vi "Write OCP Delay.vi"(8 "error in":errorcluster, 10 "Delay":dbl, 11 "3300 in":refnum<class "3300.lvclass">) -> (0 "error out":errorcluster, 3 "3300 out":refnum<class "3300.lvclass">)   [LabVIEW 2019, in "3300.lvlib" / "3300.lvclass"]
uses:
  Library/3300.lvclass
  builds/Instruments/Electronic Load.lvlibp/Library/Electronic Load.lvclass
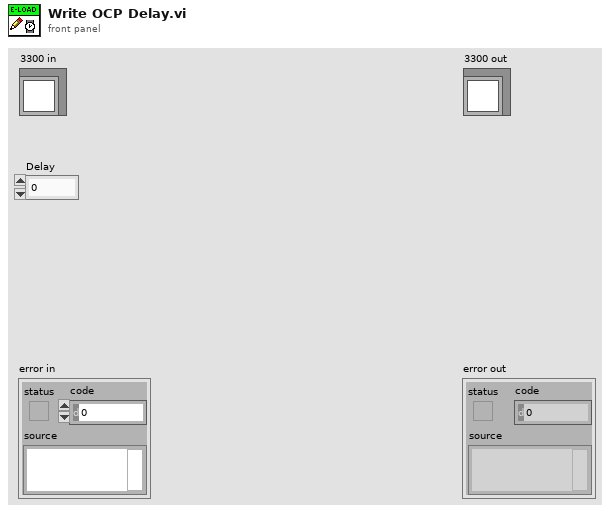
[diagram p1: front panel]
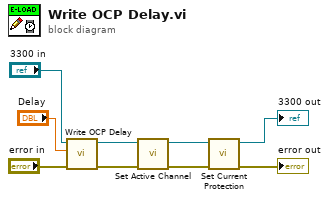
[diagram p0: block diagram]
diagram:
  n1 = call-parent "Write OCP Delay.vi"("error in"="error in", "Delay"="Delay", "Electronic Load in"="3300 in") -> ("error out"=w5:errorcluster, "Electronic Load out"=w6:refnum<class "3300.lvclass">)  [unwired: 7 in]
  n2 = call "Set Active Channel.vi"("error in"=w5, "3300 in"=w6) -> ("error out"=w3:errorcluster, "3300 out"=w4:refnum<class "3300.lvclass">)  [unwired: 8 in]
  n3 = call "Set Current Protection.vi"("error in"=w3, "3300 in"=w4) -> ("error out"=→"error out":errorcluster, "3300 out"=→"3300 out":refnum<class "3300.lvclass">)  [unwired: 8 in]
